vi "parse_project_CCSymbols.vi"(11 "CCSymbols from Project":string) -> (3 "CCSymbols":map{string, string}(c390))   [LabVIEW 2019, in "Conditional Disable Build Actions.lvlib"]
uses:
  Conditional Disable Build Actions.lvlib
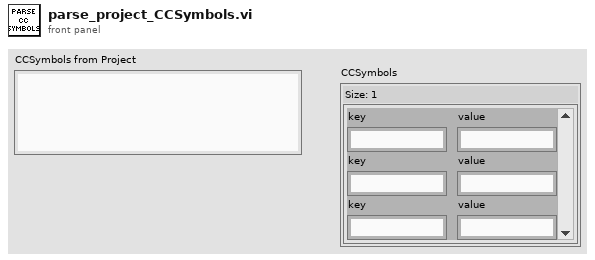
[diagram p1: front panel]
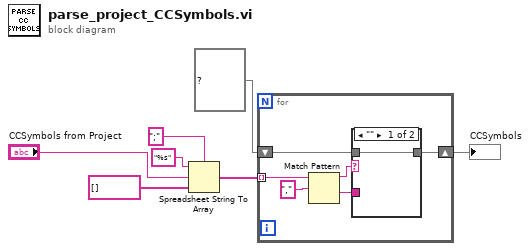
[diagram p0: block diagram]
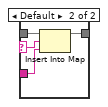
[diagram p2: hidden frame]
diagram:
  n1 = Spreadsheet String To Array(delimiter (Tab)=";", format string="%s", spreadsheet string="CCSymbols from Project", array type (2D Dbl)=string[] []) -> (array=w4:string[])
  n2 = for {
    tunnel: w4 -> [w13] mode=indexing
    shift-right: [w9] -> w2
    shift-left: map{string, string} {} ("CCSymbols") -> [w10]
    n3 = Match Pattern(string=w13, regular expression=",") -> (before substring=w8:string, after substring=w11:string)  [unwired: 1 in, 2 out]
    n4 = case shown="\"\"" w8 {
      selector: w8 -> [_ w15]
      tunnel: w11 -> [_ w18]
      tunnel: w10 -> [w14 w17]
      tunnel: [w14 w16] -> w9
      frame "" {
      }
      frame Default {
        n5 = Insert Into Map(map in=w17, key=w15, value=w18) -> (map out=w16:map{string, string})  [unwired: 2 out]
      }
    }
  }
  "CCSymbols" <- w2
